vi "统计.vi"() -> ()   [LabVIEW 2018]
panel:
  in  "停止":bool
  out "最小值":dbl
  out "最大值":dbl
  out "众数":dbl
  out "中值":dbl
  out "算术平均":dbl
  out "累加和":dbl
  out "均方根":dbl
  out "标准差":dbl
  out "方差":dbl
  in  "个数":i32
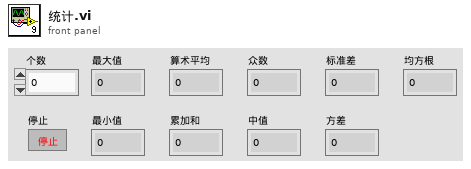
[diagram p1: front panel]
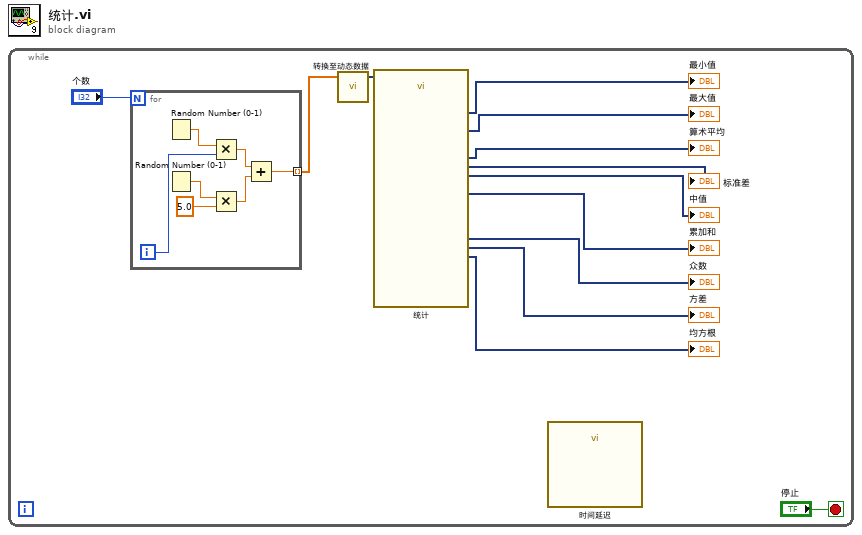
[diagram p0: block diagram]
diagram:
  n1 = while {
    stop <- "停止" stop-if-true
    n2 = for {
      N: "个数" -> [_]
      tunnel: [w14] -> w2 mode=indexing
      i -> [w17]
      n3 = Random Number (0-1)() -> (number: 0 to 1=w20:dbl)
      n4 = Random Number (0-1)() -> (number: 0 to 1=w19:dbl)
      n5 = Multiply(x=w20, y=w17) -> (x*y=w16:dbl)
      n6 = Multiply(x=w19, y=5.0) -> (x*y=w15:dbl)
      n7 = Add(x=w16, y=w15) -> (x+y=w14:dbl)
    }
    n8 = call "转换至动态数据"("Array"=w2) -> ("Dynamic Data Type"=w13:dynamicdata)  [unwired: 3 in]
    n9 = call "统计"("Signals"=w13) -> ("Summation"=→"累加和":dynamicdata, "Mode"=→"众数":dynamicdata, "Median"=→"中值":dynamicdata, "Variance"=→"方差":dynamicdata, "Standard Dev"=→"标准差":dynamicdata, "RMS"=→"均方根":dynamicdata, "Arithmetic Mean"=→"算术平均":dynamicdata, "Minimum"=→"最小值":dynamicdata, "Maximum"=→"最大值":dynamicdata)  [unwired: 4 in, 14 out]
    n10 = call "时间延迟"() -> ()  [unwired: 11 in, 1 out]
  }
